vi "Get_Configuration_Zurich.vi"(0 "Filename (.ini)":string="Config_Ver_1\\Zurich_params.ini", 11 "error in":errorcluster) -> (2 "Subscription 3":cluster{"path":string, "Channels":string[]}, 3 "Subscription 0":cluster{"path":string, "Channels":string[]}, 4 "data Acquisition Module string":T2, 6 "data Acquisition Module double":T1, 8 "general settings double":T1, 10 "general settings string":T2, 15 "error out":errorcluster)   [LabVIEW 2021]
uses:
  <vilib>/Utility/config.llb/Read Key (String).vi
  <vilib>/Utility/config.llb/Read Key (Double).vi
  <vilib>/Utility/config.llb/NI_LVConfig.lvlib
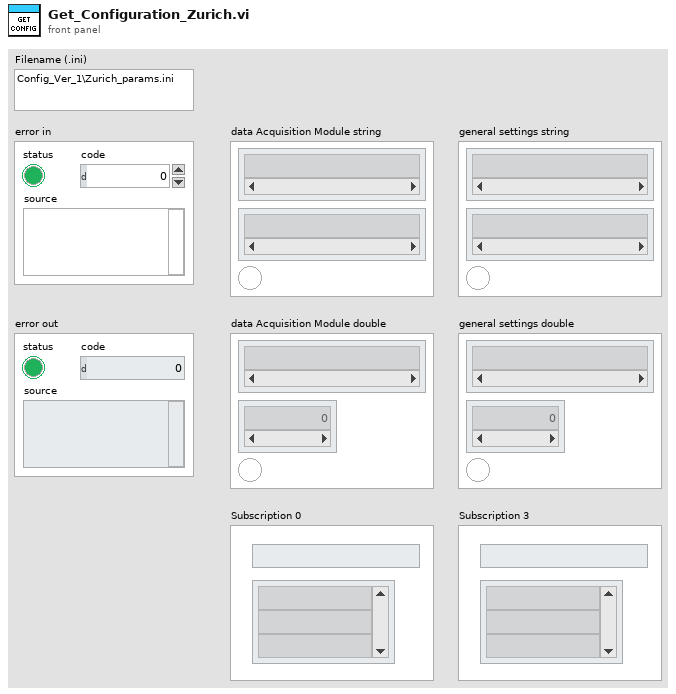
[diagram p1: front panel]
types:
  T1 = cluster{"command":string[], "value":dbl[], "section exist(?)":bool}
  T2 = cluster{"command":string[], "value":string[], "section exist(?)":bool}
  T3 = typedef "NI_LVConfig.lvlib/Config Data RefNum.ctl" = refnum<k1>
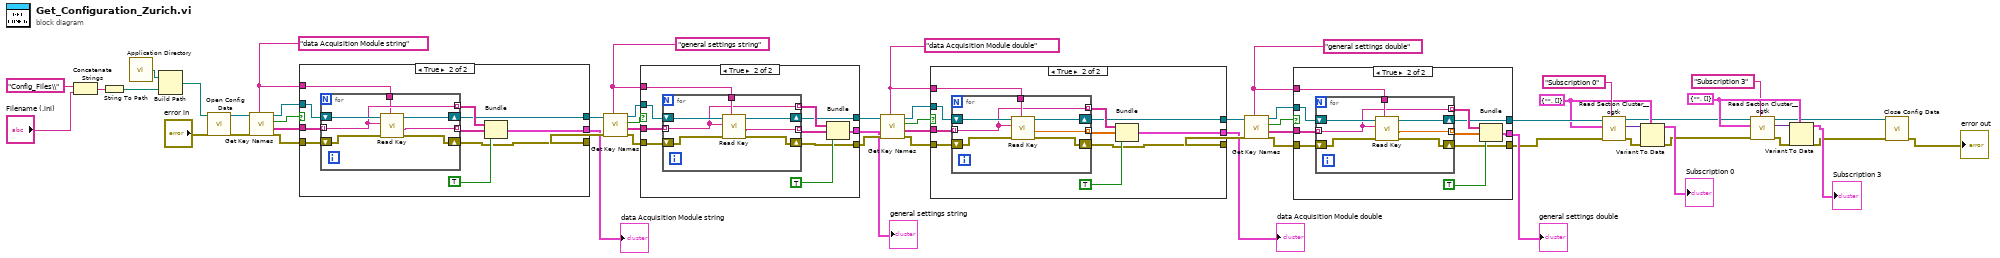
[diagram p0: block diagram]
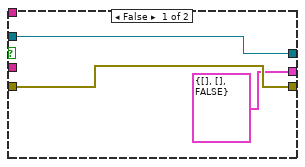
[diagram p2: hidden frame]
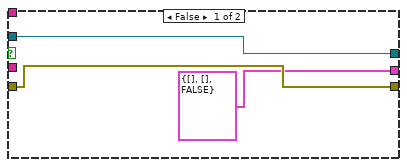
[diagram p3: hidden frame]
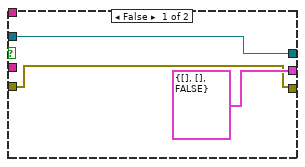
[diagram p4: hidden frame]
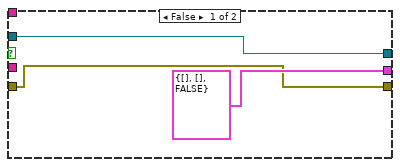
[diagram p5: hidden frame]
diagram:
  w7 = cluster{"path":string, "Channels":string[]} {"path"="", "Channels"=[]} ("Subscription")
  w14 = cluster{"path":string, "Channels":string[]} {"path"="", "Channels"=[]} ("Subscription")
  w30 = "general settings double" ("section")
  w29 = "data Acquisition Module double" ("section")
  w43 = "general settings string" ("section")
  w45 = "data Acquisition Module string" ("section")
  n1 = Concatenate Strings("Config_Files\\" ("string"), "Filename (.ini)") -> (w51:string)
  n2 = String To Path(string=w51) -> (path=w54:path)
  n3 = call <vilib>:"Application Directory.vi"() -> ("Application Directory"=w56:path)
  n4 = Build Path(base path=w56, name or relative path=w54) -> (appended path=w55:path)
  n5 = call <vilib>:"Open Config Data.vi"("error in (no error)"="error in", "configuration file path"=w55) -> ("error out"=w44:errorcluster, "refnum"=w49:T3)  [unwired: 7 in, 1 out]
  n6 = call <vilib>:"Get Key Names.vi"("section"=w45, "error in (no error)"=w44, "refnum"=w49) -> ("error out"=w47:errorcluster, "key names"=w10:string[], "section exists?"=w46:bool, "refnum out"=w48:T3)  [unwired: 5 in]
  n7 = case shown="True" w46 {
    tunnel: w48 -> [w58 w68]
    tunnel: w47 -> [w57 w69]
    tunnel: w45 -> [_ w61]
    tunnel: [cluster{string[], string[], bool} {[], [], FALSE} ("output cluster") w64] -> w22
    tunnel: [w58 w63] -> w38
    tunnel: [w57 w62] -> w37
    tunnel: w10 -> [_ w60]
    frame False {
    }
    frame True {
      n8 = for {
        tunnel: w60 -> [w71] mode=indexing
        shift-right: [w76] -> w63
        shift-left: w68 -> [w75]
        shift-right: [w73] -> w62
        shift-left: w69 -> [w74]
        tunnel: [w72] -> w66 mode=indexing
        tunnel: [w71] -> w67 mode=indexing
        tunnel: w61 -> [w70]
        n9 = call-poly <vilib>:"Read Key.vi"("section"=w70, "error in (no error)"=w74, "key"=w71, "refnum"=w75) -> ("error out"=w73:errorcluster, "value"=w72:string, "refnum out"=w76:T3)  [unwired: 4 in, 1 out]
      }
      n10 = Bundle(w67, w66, TRUE) -> (w64:cluster{string[], string[], bool})  [unwired: 1 in]
    }
  }
  "data Acquisition Module string" <- w22
  n11 = call <vilib>:"Get Key Names.vi"("section"=w43, "error in (no error)"=w37, "refnum"=w38) -> ("error out"=w41:errorcluster, "key names"=w39:string[], "section exists?"=w42:bool, "refnum out"=w40:T3)  [unwired: 5 in]
  n12 = case shown="True" w42 {
    tunnel: w39 -> [_ w89]
    tunnel: w40 -> [w78 w87]
    tunnel: w41 -> [w77 w88]
    tunnel: w43 -> [_ w86]
    tunnel: [cluster{string[], string[], bool} {[], [], FALSE} ("output cluster") w82] -> w21
    tunnel: [w78 w81] -> w24
    tunnel: [w77 w80] -> w23
    frame False {
    }
    frame True {
      n13 = for {
        tunnel: w89 -> [w90] mode=indexing
        shift-right: [w96] -> w81
        shift-left: w87 -> [w95]
        shift-right: [w93] -> w80
        shift-left: w88 -> [w94]
        tunnel: w86 -> [w91]
        tunnel: [w92] -> w84 mode=indexing
        tunnel: [w90] -> w85 mode=indexing
        n14 = call-poly <vilib>:"Read Key.vi"("section"=w91, "error in (no error)"=w94, "key"=w90, "refnum"=w95) -> ("error out"=w93:errorcluster, "value"=w92:string, "refnum out"=w96:T3)  [unwired: 4 in, 1 out]
      }
      n15 = Bundle(w85, w84, TRUE) -> (w82:cluster{string[], string[], bool})  [unwired: 1 in]
    }
  }
  "general settings string" <- w21
  n16 = call <vilib>:"Get Key Names.vi"("section"=w29, "error in (no error)"=w23, "refnum"=w24) -> ("error out"=w27:errorcluster, "key names"=w25:string[], "section exists?"=w28:bool, "refnum out"=w26:T3)  [unwired: 5 in]
  n17 = case shown="True" w28 {
    tunnel: w25 -> [_ w109]
    tunnel: w26 -> [w99 w107]
    tunnel: w27 -> [w98 w108]
    tunnel: w29 -> [_ w106]
    tunnel: [w99 w102] -> w35
    tunnel: [w98 w101] -> w36
    tunnel: [cluster{string[], dbl[], bool} {[], [], FALSE} ("output cluster") w100] -> w20
    frame False {
    }
    frame True {
      n18 = for {
        tunnel: w109 -> [w110] mode=indexing
        shift-right: [w116] -> w102
        shift-left: w107 -> [w115]
        shift-right: [w113] -> w101
        shift-left: w108 -> [w114]
        tunnel: w106 -> [w111]
        tunnel: [w112] -> w104 mode=indexing
        tunnel: [w110] -> w105 mode=indexing
        n19 = call-poly <vilib>:"Read Key.vi"("section"=w111, "error in (no error)"=w114, "key"=w110, "refnum"=w115) -> ("error out"=w113:errorcluster, "value"=w112:dbl, "refnum out"=w116:T3)  [unwired: 4 in, 1 out]
      }
      n20 = Bundle(w105, w104, TRUE) -> (w100:cluster{string[], dbl[], bool})  [unwired: 1 in]
    }
  }
  "data Acquisition Module double" <- w20
  n21 = call <vilib>:"Get Key Names.vi"("section"=w30, "error in (no error)"=w36, "refnum"=w35) -> ("error out"=w32:errorcluster, "key names"=w34:string[], "section exists?"=w31:bool, "refnum out"=w33:T3)  [unwired: 5 in]
  n22 = case shown="True" w31 {
    tunnel: w34 -> [_ w129]
    tunnel: w33 -> [w119 w127]
    tunnel: w32 -> [w118 w128]
    tunnel: w30 -> [_ w126]
    tunnel: [w119 w122] -> w17
    tunnel: [w118 w121] -> w16
    tunnel: [cluster{string[], dbl[], bool} {[], [], FALSE} ("output cluster") w120] -> w19
    frame False {
    }
    frame True {
      n23 = for {
        tunnel: w129 -> [w130] mode=indexing
        shift-right: [w136] -> w122
        shift-left: w127 -> [w135]
        shift-right: [w133] -> w121
        shift-left: w128 -> [w134]
        tunnel: w126 -> [w131]
        tunnel: [w132] -> w124 mode=indexing
        tunnel: [w130] -> w125 mode=indexing
        n24 = call-poly <vilib>:"Read Key.vi"("section"=w131, "error in (no error)"=w134, "key"=w130, "refnum"=w135) -> ("error out"=w133:errorcluster, "value"=w132:dbl, "refnum out"=w136:T3)  [unwired: 4 in, 1 out]
      }
      n25 = Bundle(w125, w124, TRUE) -> (w120:cluster{string[], dbl[], bool})  [unwired: 1 in]
    }
  }
  "general settings double" <- w19
  n26 = call <userlib>:"Read Section Cluster__ogtk.vi"("section (optional)"="Subscription 0", "error in (no error)"=w16, "Section Formatted Cluster Type"=w14, "refnum"=w17) -> ("error out"=w12:errorcluster, "Section Formatted Cluster"=w13:variant, "dup refnum"=w5:T3)  [unwired: 3 in, 2 out]
  n27 = Variant To Data(error in=w12, type=w14, Variant=w13) -> (data=→"Subscription 0":cluster{"path":string, "Channels":string[]}, error out=w4:errorcluster)
  n28 = call <userlib>:"Read Section Cluster__ogtk.vi"("section (optional)"="Subscription 3", "error in (no error)"=w4, "Section Formatted Cluster Type"=w7, "refnum"=w5) -> ("error out"=w9:errorcluster, "Section Formatted Cluster"=w8:variant, "dup refnum"=w2:T3)  [unwired: 3 in, 2 out]
  n29 = Variant To Data(error in=w9, type=w7, Variant=w8) -> (data=→"Subscription 3":cluster{"path":string, "Channels":string[]}, error out=w1:errorcluster)
  n30 = call <vilib>:"Close Config Data.vi"("error in (no error)"=w1, "refnum"=w2) -> ("error out"=→"error out":errorcluster)  [unwired: 8 in, 1 out]
